vi "Aggregate.vi"(7 "ModuleAdmin":refnum<class "ModuleAdmin.lvclass">, 8 "error in (no error)":errorcluster, 11 "AppPluginsBase in":refnum<class "AppPluginsBase.lvclass">) -> (0 "error out":errorcluster, 3 "AppPluginsBase out":refnum<class "AppPluginsBase.lvclass">)   [LabVIEW 2017, in "AppPlugins.lvlib" / "AppPluginsBase.lvclass"]
uses:
  AppPluginsBase.lvclass
  <userlib>/NIST/ModuleAdminLib/ModuleAdmin/ModuleAdmin.lvclass
  Framework/BusController/Queue/QueueType.ctl
  EventPlugins/EventPluginBaseClass/TypeDefs/clEvtReportArray.ctl
  EventPlugins/EventPluginBaseClass/TypeDefs/clEvtReport.ctl
  AppPluginsBase.lvclass/AppPluginsBase.ctl
  Framework/Bus_class/Public/TypeDefs/clBusData.ctl
  Framework/FrontPanel/TypeDefs/clEventConfig.ctl
  PmuImpairPlugins/PmuImpairPluginBase_class/TypeDefs/clImpairConfig.ctl
  EventPlugins/EventPluginBaseClass/TypeDefs/dblEvtSignalArray.ctl
  NetworkImpairmentModule/PublicAPI/Arguments/Broadcasts/dblNetworkTime.ctl
  NetworkImpairmentModule/PublicAPI/Arguments/Broadcasts/dblPktLoss.ctl
  FlagImpairModule/PublicAPI/Arguments/Broadcasts/ui32FlagImpairmentArray.ctl
  OutputToFilePlugins/OutputToFileBasePlugin/Typedefs/PmuCfgOpt.ctl
  Accessors/Read BC_AppInfo.vi
  Accessors/Write clEvtReportArray.vi
  <vilib>/Utility/error.llb/Error Cluster From Error Code.vi
  Framework/BusController/Admin/Registry/BCReg.lvclass
  <vilib>/ErrorRing/Error Ring.xnode
  AppModule/AppModule.lvlib
  Framework/BusController/BusController.lvlib
  Framework/Framework.lvlib
  PmuImpairPlugins/PmuImpairPluginBase_class/PmuImpairPluginBase.lvclass
  EventPlugins/EventPluginBaseClass/EventPluginBaseClass.lvclass
  NetworkImpairmentModule/NetworkImpairmentModule.lvlib
  FlagImpairModule/FlagImpairModule.lvlib
  OutputToFilePlugins/OutputToFileBasePlugin/OutputToFileBasePlugin.lvclass
  Framework/Bus_class/Bus.lvclass
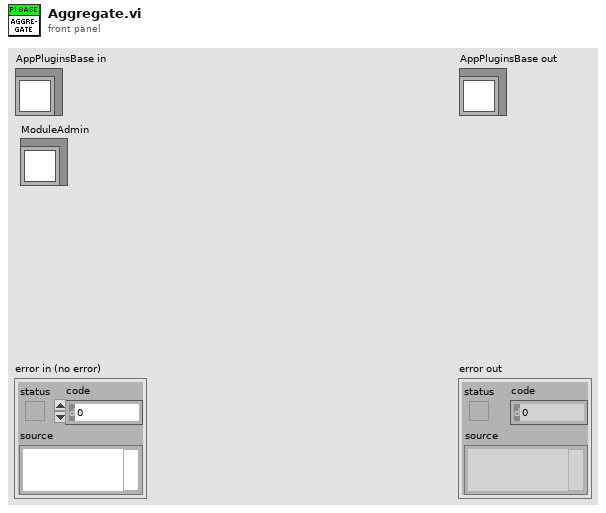
[diagram p1: front panel]
types:
  T1 = typedef "EventPlugins.lvlib/EventPluginBaseClass.lvclass/clEvtReportArray.ctl" = T2[]
  T2 = typedef "EventPlugins.lvlib/EventPluginBaseClass.lvclass/clEvtReport.ctl" = cluster{"Timestamp":dbl, "Synx":cdb[], "Freq":dbl, "ROCOF":dbl, "ID":i16}
  T3 = typedef "BusController.lvlib/QueueType.ctl" = cluster{"Msg":string, "Data":variant}
  T4 = typedef "Bus_class.lvlib/Bus.lvclass/clBusData.ctl" = cluster{"BusNumber":u8, "EvtPluginINIFilePath":path, "EvtParams":string[][], "EvtConfig":T5, "Start Time":dbl, "End Time":dbl, "PmuImpairPluginINIFilePath":path, "PmuImpairParams ":string[][], "PmuImpairConfig":T6, "NetImpPluginINIFilePath":path, "NetImpParams":string[][], "FlagImpPluginINIFilePath":path, "FlagImpParams":string[][], "EvtReportArray":T1, "EventSignalArray":T7, "ImpairReportArray":T1, "NetworkTime":T8, "PktLoss":T9, "FlagImpArray":T10, "OutputToFilePluginINIFilePath":path, "Output File Path":path, "clConfigOptions":T11, "AppPluginINIFilePath":path, "AppConfig":variant, "AppOutput":variant}
  T5 = typedef "Framework.lvlib/clEventConfig.ctl" = cluster{"UTC Time 0":timestamp, "Nominal Frequency":u16, "Reporting Rate":u16, "Fsamp":u32, "PosSeq":bool}
  T6 = typedef "PmuImpairPlugins.lvlib/PmuImpairPluginBase.lvclass/clImpairConfig.ctl" = cluster{"FilterType":string, "bPosSeq":bool}
  T7 = typedef "EventPlugins.lvlib/EventPluginBaseClass.lvclass/dblEvtSignalArray.ctl" = dbl[][]
  T8 = typedef "NetworkImpairmentModule.lvlib/dblNetworkTime.ctl" = dbl[]
  T9 = typedef "NetworkImpairmentModule.lvlib/dblPktLoss.ctl" = dbl[]
  T10 = typedef "FlagImpairModule.lvlib/ui32FlagImpairmentArray.ctl" = u32[]
  T11 = typedef "OutputToFilePlugins.lvlib/OutputToFileBasePlugin.lvclass/PmuCfgOpt.ctl" = cluster{"TIME_BASE":u64, "STN":string, "IDCODE":u16, "rdoPolRect":enum32{"Rectangular", "Polar"}, "rdoFloatInt":enum32{"Float", "Integer"}, "PHUNIT":u64, "rdoFreqDfreq":enum32{"Float", "Integer"}, "CHNAM":string[], "chkCfg2Prefix":bool}
  T12 = typedef "AppModule.lvlib/BC_AppInfo.ctl" = cluster{"QueName":string, "BCRegRef":refnum<data-value>}
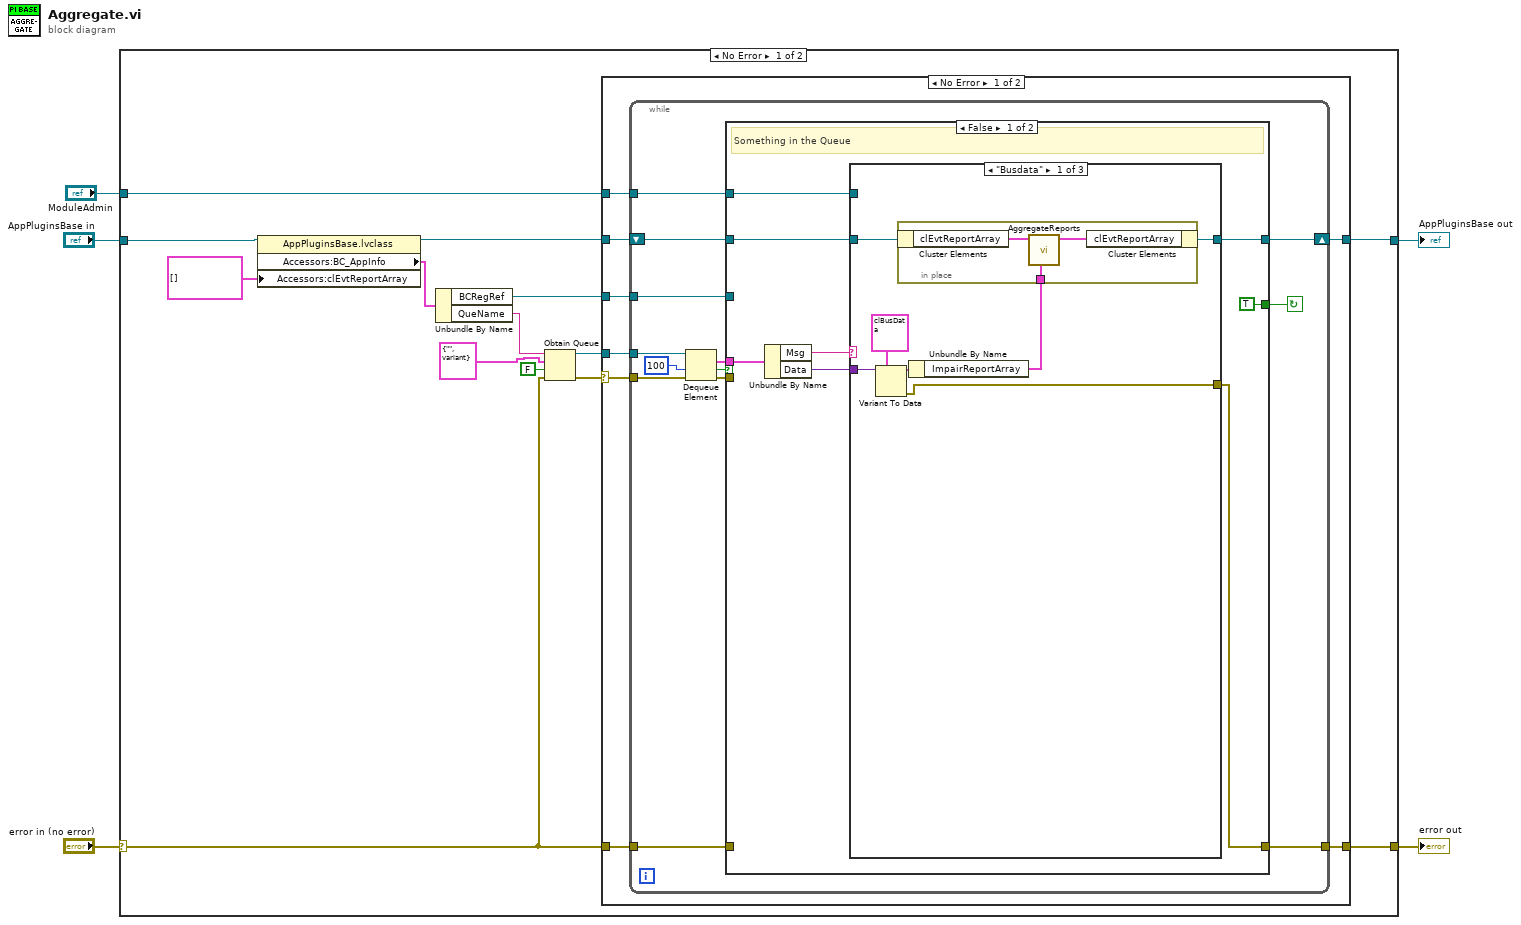
[diagram p0: block diagram]
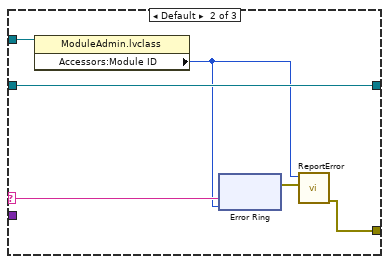
[diagram p2: hidden frame]
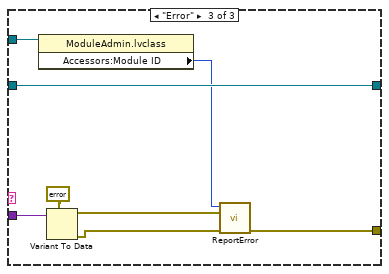
[diagram p3: hidden frame]
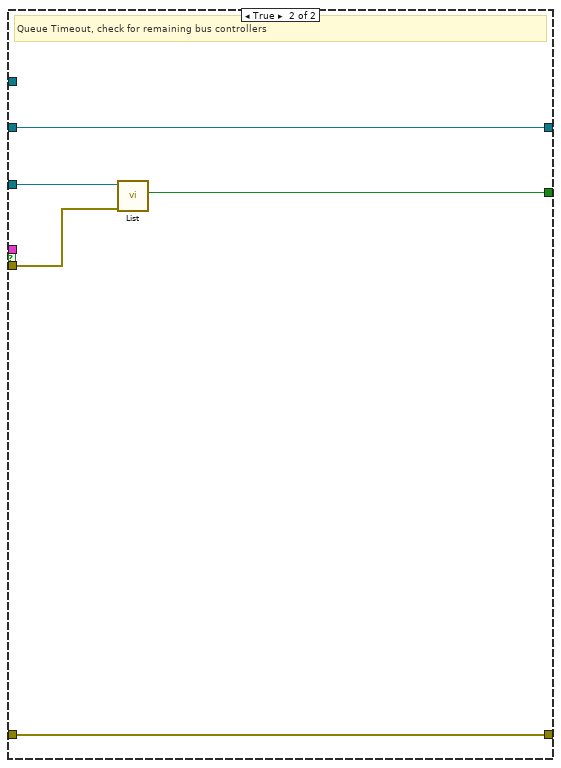
[diagram p4: hidden frame]
diagram:
  n1 = case shown="No Error" "error in (no error)" {
    selector: "error in (no error)" -> [w15 w89]
    tunnel: [w12 w89] -> w4
    tunnel: [w9 w88] -> w2
    tunnel: "AppPluginsBase in" -> [w19 w88]
    tunnel: "ModuleAdmin" -> [w8 _]
    frame No Error {
      n2 = property class="AppPluginsBase.lvclass"(reference=w19, "Accessors:clEvtReportArray"=T1 [] ("clEvtReportArray")) -> (reference out=w10:refnum<class "AppPluginsBase.lvclass">, "Accessors:BC_AppInfo"=w18:T12)  [unwired: 1 in, 1 out]
      n3 = Unbundle By Name(w18) -> ("BCRegRef"=w11:refnum<data-value>, "QueName"=w17:string)
      n4 = Obtain Queue(name (unnamed)=w17, element data type=T3 {"Msg"="", "Data"=variant} ("QueueType"), create if not found? (T)=FALSE, error in (no error)=w15) -> (queue out=w13:refnum<queue>, error out=w14:errorcluster)  [unwired: 1 in, 1 out]
      n5 = case shown="No Error" w14 {
        selector: w14 -> [w25 w87]
        tunnel: w15 -> [w27 _]
        tunnel: w13 -> [w24 _]
        tunnel: [w26 w87] -> w12
        tunnel: w11 -> [w23 _]
        tunnel: w10 -> [w22 w86]
        tunnel: [w21 w86] -> w9
        tunnel: w8 -> [w20 _]
        frame No Error {
          n6 = while {
            tunnel: w27 -> [w30]
            tunnel: [w29] -> w26
            tunnel: w25 -> [w40]
            tunnel: w24 -> [w39]
            tunnel: w23 -> [w36]
            shift-right: [w34] -> w21
            shift-left: w22 -> [w35]
            tunnel: w20 -> [w28]
            stop <- w31 continue-if-true
            n7 = Dequeue Element(queue=w39, timeout in ms (-1)=100, error in (no error)=w40) -> (element=w32:T3, timed out?=w37:bool, error out=w33:errorcluster)  [unwired: 1 out]
            n8 = case shown="False" w37 {
              tunnel: w36 -> [_ w84]
              tunnel: w35 -> [w44 w85]
              tunnel: [w42 w85] -> w34
              tunnel: w33 -> [_ w82]
              tunnel: w32 -> [w47 _]
              tunnel: [TRUE w83] -> w31
              tunnel: w30 -> [_ w81]
              tunnel: [w41 w81] -> w29
              tunnel: w28 -> [w43 _]
              frame False {
                # "Something in the Queue"
                n9 = Unbundle By Name(w47) -> ("Msg"=w46:string, "Data"=w45:variant)
                n10 = case shown="\"Busdata\"" w46 {
                  selector: w46 -> [_ w60 _]
                  tunnel: w45 -> [w55 _ w80]
                  tunnel: w44 -> [w53 w61 w77]
                  tunnel: w43 -> [_ w64 w78]
                  tunnel: [w50 w61 w77] -> w42
                  tunnel: [w49 w62 w73] -> w41
                  frame "Busdata" {
                    n11 = Variant To Data(type=T4 {"BusNumber"=0, "EvtPluginINIFilePath"=path "", "EvtParams"=[], "EvtConfig"={"UTC Time 0"=timestamp(0 s since 1904-01-01), "Nominal Frequency"=60, "Reporting Rate"=60, "Fsamp"=960, "PosSeq"=FALSE}, "Start Time"=0.0, "End Time"=0.0, "PmuImpairPluginINIFilePath"=path "", "PmuImpairParams "=[["960"], ["8.19"], ["164"]], "PmuImpairConfig"={"FilterType"="", "bPosSeq"=TRUE}, "NetImpPluginINIFilePath"=path "", "NetImpParams"=[], "FlagImpPluginINIFilePath"=path "", "FlagImpParams"=[], "EvtReportArray"=[], "EventSignalArray"=[], "ImpairReportArray"=[], "NetworkTime"=[], "PktLoss"=[], "FlagImpArray"=[], "OutputToFilePluginINIFilePath"=path "", "Output File Path"=path "", "clConfigOptions"={"TIME_BASE"=1000000, "STN"="Bus_1", "IDCODE"=0, "rdoPolRect"=enum."Rectangular", "rdoFloatInt"=enum."Float", "PHUNIT"=1000000, "rdoFreqDfreq"=enum."Float", "CHNAM"=["VA", "VB", "VC", "V+", "IA", "IB", "IC", "I+"], "chkCfg2Prefix"=TRUE}, "AppPluginINIFilePath"=path "", "AppConfig"=variant, "AppOutput"=variant} ("clBusData"), Variant=w55) -> (data=w52:T4, error out=w49:errorcluster)  [unwired: 1 in]
                    n12 = Unbundle By Name(w52) -> ("ImpairReportArray"=w51:T1)
                    n13 = in-place {
                      in-place-border: w51 -> [w56]
                      n14 = in-place-cluster #1(w53) -> ("clEvtReportArray"=w58:T1)
                      n15 = call "AggregateReports.vi"("Additional In"=w56, "Aggregated In"=w58) -> ("Aggregated Out"=w57:T1)  [unwired: 9 in]
                      n16 = in-place-cluster #1("clEvtReportArray"=w57) -> (w50:refnum<class "AppPluginsBase.lvclass">)
                    }
                  }
                  frame Default {
                    n17 = property class="ModuleAdmin.lvclass"(reference=w64) -> ("Accessors:Module ID"=w59:i32)  [unwired: 1 in, 2 out]
                    n18 = xnode ("Error Ring")("parameter 0"=w60, "parameter 1"=w59) -> ("error out"=w63:errorcluster)
                    n19 = call "ReportError.vi"("ErrorReported"=w63, "ModuleID"=w59) -> ("error out"=w62:errorcluster)  [unwired: 9 in]
                  }
                  frame "Error" {
                    n20 = property class="ModuleAdmin.lvclass"(reference=w78) -> ("Accessors:Module ID"=w76:i32)  [unwired: 1 in, 2 out]
                    n21 = Variant To Data(type=errorcluster {"status"=FALSE, "code"=0, "source"=""} ("error constant"), Variant=w80) -> (data=w75:errorcluster, error out=w74:errorcluster)  [unwired: 1 in]
                    n22 = call "ReportError.vi"("error in (no error)"=w74, "ErrorReported"=w75, "ModuleID"=w76) -> ("error out"=w73:errorcluster)  [unwired: 8 in]
                  }
                }
              }
              frame True {
                # "Queue Timeout, check for remaining bus controllers"
                n23 = call "List.vi"("error in (no error)"=w82, "BCReg"=w84) -> ("Found?"=w83:bool)  [unwired: 4 in, 5 out]
              }
            }
          }
        }
        frame Error {
        }
      }
    }
    frame Error {
    }
  }
  "error out" <- w4
  "AppPluginsBase out" <- w2
